vi "Robot Main.vi"() -> ()   [LabVIEW 2012]
doc: "This VI imlements the framework and scheduler for your robotics program. It should not be necessary to modify the framework. You are expected to add your code to the VIs called from Robot Main, the ones located in the Team Code within the project."
uses:
  Robot Global Data.vi
panel:
  in  "Finish":bool
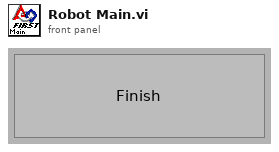
[diagram p1: front panel]
types:
  T1 = typedef "WPI_DriverStationMatch Info.ctl" = cluster{"Autonomous Elapsed Seconds":dbl, "TeleOp Elapsed Seconds":dbl, "Disabled Elapsed Seconds":dbl, "Visited Autonomous":bool, "Visited TeleOp":bool, "Visited Disabled":bool, "Autonomous Settings":cluster{"Autonomous Style":enum16{"Iterative", "Independent"}, "VI Refnum":refnum<vi>}}
  T2 = typedef "WPI_DriverStationDerivedRobotMode.ctl" = enum16{"Init", "Execute", "Stop"}
  T3 = typedef "WPI_DriverStationRobotMode2.ctl" = enum16{"Autonomous Disabled", "Autonomous Enabled", "Teleop Disabled", "Teleop Enabled", "Timeout", "Finish", "Test Disabled", "Test Enabled"}
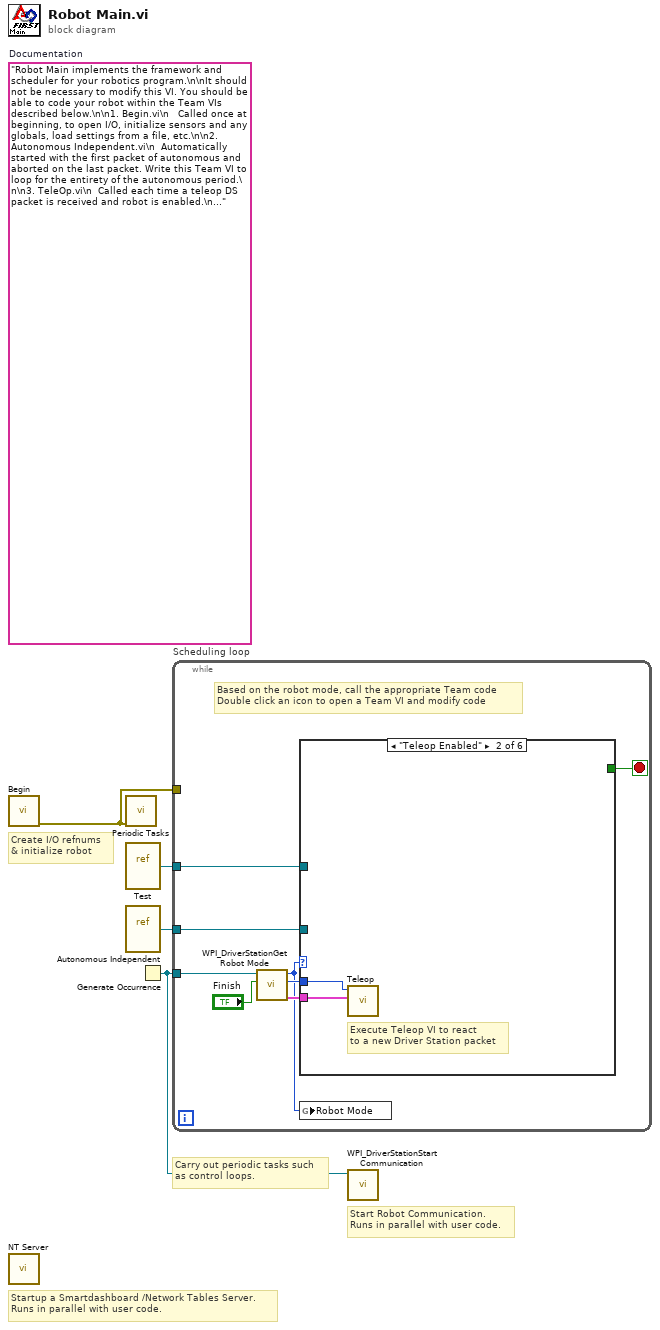
[diagram p0: block diagram]
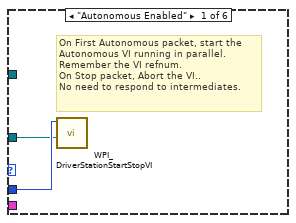
[diagram p2: hidden frame]
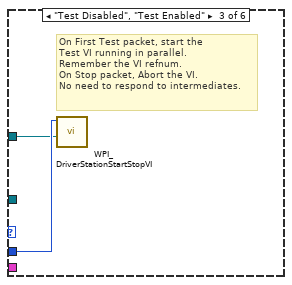
[diagram p3: hidden frame]
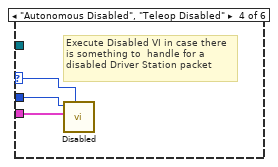
[diagram p4: hidden frame]
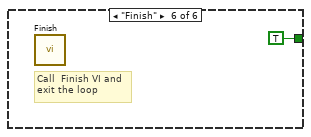
[diagram p6: hidden frame]
diagram:
  (unwired) "Robot Main implements the framework and scheduler for your robotics program.\n\nIt should not be necessary to modify this VI. You should be able to code your robot within the Team VIs described below.\n\n1. Begin.vi\n   Called once at beginning, to open I/O, initialize sensors and any globals, load settings from a file, etc.\n\n2. Autonomous Independent.vi\n  Automatically started with the first packet of autonomous and aborted on the last packet. Write this Team VI to loop for the entirety of the autonomous period.\n\n3. TeleOp.vi\n  Called each time a teleop DS packet is received and robot is enabled.\n\n4. Disabled.vi\n  Called each time a packet is received and the robot is disabled.\n\n5. Test.vi\n  Called Automatically started with the first test packet and aborted on the last. Modify this VI to carry out robot and sensor validation tests.\n\n6. Vision.vi\n  A parallel loop that acquires and processes camera images.\n\n7. PeriodicTasks.vi\n  Parallel loops running at user-defined rates.\n\n8. Finish.vi\n  Called before exiting, so you can save data, clean up I/O, etc.\n"  # Documentation
  # "Startup a Smartdashboard /Network Tables Server.\nRuns in parallel with user code."
  # "Carry out periodic tasks such\nas control loops."
  # "Create I/O refnums\n& initialize robot"
  # "Start Robot Communication.\nRuns in parallel with user code."
  n1 = call "Begin.vi"() -> ("error out"=w2:errorcluster)  [unwired: 1 in, 10 out]
  n2 = call <vilib>:"NT Server.vi"() -> ()  [unwired: 12 in]
  n3 = call "Periodic Tasks.vi"("error in"=w2) -> ()  [unwired: 1 in, 10 out]
  n4 = vi-ref "Test.vi"() -> (w1:refnum<vi>)
  n5 = vi-ref "Autonomous Independent.vi"() -> (w3:refnum<vi>)
  n6 = Generate Occurrence() -> (w4:refnum<k4>)
  n7 = while "Scheduling loop" {
    tunnel: w4 -> [w11]
    tunnel: w2 -> [_]
    tunnel: w3 -> [w7]
    tunnel: w1 -> [w6]
    stop <- w8 stop-if-true
    # "Based on the robot mode, call the appropriate Team code\nDouble click an icon to open a Team VI and modify code"
    n8 = call <vilib>:"WPI_DriverStationGet Robot Mode.vi"("Finish"="Finish", "DS Occurrence"=w11) -> ("Match Info out"=w9:T1, "Call Context"=w12:T2, "Robot Mode"=w5:T3)  [unwired: 7 out]
    n9 = case shown="\"Teleop Enabled\"" w5 {
      selector: w5 -> [_ _ _ w19 _ _]
      tunnel: w12 -> [w14 w16 w18 w21 _ _]
      tunnel: w9 -> [_ w15 _ w20 _ _]
      tunnel: [_ _ _ _ _ TRUE] -> w8
      tunnel: w7 -> [w13 _ _ _ _ _]
      tunnel: w6 -> [_ _ w17 _ _ _]
      frame "Autonomous Enabled" {
        # "On First Autonomous packet, start the\nAutonomous VI running in parallel.\nRemember the VI refnum.\nOn Stop packet, Abort the VI..\nNo need to respond to intermediates."
        n10 = call <vilib>:"WPI_DriverStationStartStopVI.vi"("VI in"=w13, "Call Context"=w14) -> ()  [unwired: 10 in]
      }
      frame "Teleop Enabled" {
        # "Execute Teleop VI to react\nto a new Driver Station packet"
        n11 = call "Teleop.vi"("Match Info"=w15, "Call Context"=w16) -> ()  [unwired: 1 in, 9 out]
      }
      frame "Test Disabled", "Test Enabled" {
        # "On First Test packet, start the\nTest VI running in parallel.\nRemember the VI refnum.\nOn Stop packet, Abort the VI.\nNo need to respond to intermediates."
        n12 = call <vilib>:"WPI_DriverStationStartStopVI.vi"("VI in"=w17, "Call Context"=w18) -> ()  [unwired: 10 in]
      }
      frame "Autonomous Disabled", "Teleop Disabled" {
        # "Execute Disabled VI in case there\nis something to  handle for a\ndisabled Driver Station packet"
        n13 = call "Disabled.vi"("Robot Mode"=w19, "Match Info"=w20, "Call Context"=w21) -> ()  [unwired: 1 in, 8 out]
      }
      frame "Timeout" {
        # "Driver Station packet didn't arrive.\nPossibly useful for diagnostics"
      }
      frame "Finish" {
        # "Call  Finish VI and\nexit the loop"
        n14 = call "Finish.vi"() -> ()  [unwired: 1 in, 7 out]
      }
    }
    n15 = global write "Robot Global Data.vi" "Robot Mode"(w5) -> ()
  }
  n16 = call <vilib>:"WPI_DriverStationStart Communication.vi"("occurrence"=w4) -> ()  [unwired: 11 out]
